vi "TestCases.vi"() -> ()   [LabVIEW 2020]
uses:
  JKISM++ API String Arguments Support.lvlib
panel:
  in  "String 9":string="Name:abc;child.name:ddd"
  out "error 9":errorcluster
  out "Data 8":T1={"Name"="abc", "Child"={"Name"=""}, "Bool"=TRUE}
  in  "String 8":string="[3.12,4.11,5]"
  out "error 8":errorcluster
  out "Data 4":dbl[](array[numeric])=[3.12, 4.11, 5.0]
  in  "String 7":string="ccccc"
  out "error 7":errorcluster
  out "Data 7":enum16{"1 - aaaa", "2 - bbbb", "555 - ccccc"}(ring)=enum."555 - ccccc"
  in  "String 6":string="555"
  out "error 6":errorcluster
  out "Data 6":enum16{"1 - aaaa", "2 - bbbb", "555 - ccccc"}(ring)=enum."555 - ccccc"
  in  "String 5":string="bbbb"
  out "error 5":errorcluster
  out "Data 5":enum16{"aaaa", "bbbb", "ccccc"}(ring)=enum."bbbb"
  in  "String 4":string="3.1415926"
  out "error 4":errorcluster
  out "Data 4":dbl=3.1415926
  in  "String 3":string="0x42"
  out "error 3":errorcluster
  out "Data 3":i32=66
  in  "String 2":string="Enable"
  out "error 2":errorcluster
  out "Data 2":bool=TRUE
  out "Data 1":string="abcd"
  out "error 1":errorcluster
  in  "String":string="abcd"
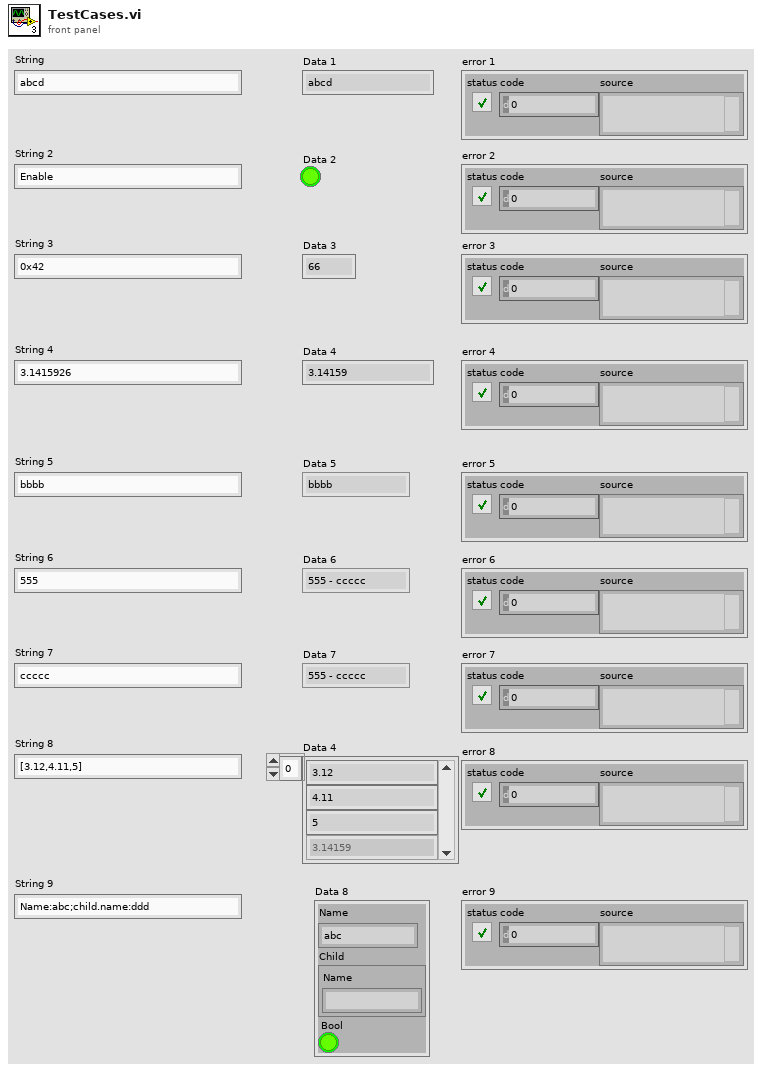
[diagram p1: front panel]
types:
  T1 = cluster{"Name":string, "Child":cluster{"Name":string}, "Bool":bool}
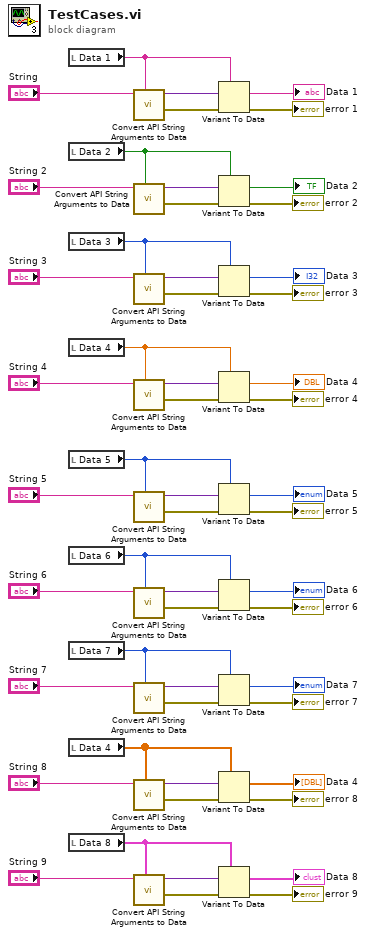
[diagram p0: block diagram]
diagram:
  n1 = local read "Data 1"() -> (w52:string)
  n2 = local read "Data 2"() -> (w51:bool)
  n3 = local read "Data 3"() -> (w46:i32)
  n4 = local read "Data 4"() -> (w45:dbl)
  n5 = local read "Data 5"() -> (w40:enum16{"aaaa", "bbbb", "ccccc"})
  n6 = local read "Data 6"() -> (w39:enum16{"1 - aaaa", "2 - bbbb", "555 - ccccc"})
  n7 = local read "Data 7"() -> (w34:enum16{"1 - aaaa", "2 - bbbb", "555 - ccccc"})
  n8 = local read "Data 4"() -> (w33:dbl[])
  n9 = local read "Data 8"() -> (w28:T1)
  n10 = call "Convert API String Arguments to Data.vi"("Type"=w52, "String"="String") -> ("error"=w2:errorcluster, "Data"=w3:variant)  [unwired: 8 in]
  n11 = call "Convert API String Arguments to Data.vi"("Type"=w51, "String"="String 2") -> ("error"=w26:errorcluster, "Data"=w25:variant)  [unwired: 8 in]
  n12 = call "Convert API String Arguments to Data.vi"("Type"=w46, "String"="String 3") -> ("error"=w23:errorcluster, "Data"=w24:variant)  [unwired: 8 in]
  n13 = call "Convert API String Arguments to Data.vi"("Type"=w45, "String"="String 4") -> ("error"=w21:errorcluster, "Data"=w22:variant)  [unwired: 8 in]
  n14 = call "Convert API String Arguments to Data.vi"("Type"=w40, "String"="String 5") -> ("error"=w19:errorcluster, "Data"=w20:variant)  [unwired: 8 in]
  n15 = call "Convert API String Arguments to Data.vi"("Type"=w39, "String"="String 6") -> ("error"=w17:errorcluster, "Data"=w18:variant)  [unwired: 8 in]
  n16 = call "Convert API String Arguments to Data.vi"("Type"=w34, "String"="String 7") -> ("error"=w15:errorcluster, "Data"=w16:variant)  [unwired: 8 in]
  n17 = call "Convert API String Arguments to Data.vi"("Type"=w33, "String"="String 8") -> ("error"=w13:errorcluster, "Data"=w14:variant)  [unwired: 8 in]
  n18 = call "Convert API String Arguments to Data.vi"("Type"=w28, "String"="String 9") -> ("error"=w11:errorcluster, "Data"=w12:variant)  [unwired: 8 in]
  n19 = Variant To Data(error in=w2, type=w52, Variant=w3) -> (data=→"Data 1":string, error out=→"error 1":errorcluster)
  n20 = Variant To Data(error in=w26, type=w51, Variant=w25) -> (data=→"Data 2":bool, error out=→"error 2":errorcluster)
  n21 = Variant To Data(error in=w23, type=w46, Variant=w24) -> (data=→"Data 3":i32, error out=→"error 3":errorcluster)
  n22 = Variant To Data(error in=w21, type=w45, Variant=w22) -> (data=→"Data 4":dbl, error out=→"error 4":errorcluster)
  n23 = Variant To Data(error in=w19, type=w40, Variant=w20) -> (data=→"Data 5":enum16{"aaaa", "bbbb", "ccccc"}, error out=→"error 5":errorcluster)
  n24 = Variant To Data(error in=w17, type=w39, Variant=w18) -> (data=→"Data 6":enum16{"1 - aaaa", "2 - bbbb", "555 - ccccc"}, error out=→"error 6":errorcluster)
  n25 = Variant To Data(error in=w15, type=w34, Variant=w16) -> (data=→"Data 7":enum16{"1 - aaaa", "2 - bbbb", "555 - ccccc"}, error out=→"error 7":errorcluster)
  n26 = Variant To Data(error in=w13, type=w33, Variant=w14) -> (data=→"Data 4":dbl[], error out=→"error 8":errorcluster)
  n27 = Variant To Data(error in=w11, type=w28, Variant=w12) -> (data=→"Data 8":T1, error out=→"error 9":errorcluster)
